vi "ControlArmInterface.vi"() -> ()   [LabVIEW 2024]
uses:
  <vilib>/Instr/_visa.llb/VISA Configure Serial Port (Instr).vi
panel:
  out "string":string
  in  "Power Button":bool
  in  "Position Maximum":bool
  in  "Position Minimum":bool
  in  "BackwardButton":bool
  in  "ForwardButton":bool
  in  "ScramButton":bool
  in  "SpeedSelectButton":bool
  in  "ElectormagnetButton":bool
  out "Analog In 4":u16(slide)=187 scale=0.0..1023.0
  out "Analog In 3":u16(slide)=187 scale=0.0..1023.0
  out "Analog In 2":u16(slide)=187 scale=0.0..1023.0
  out "Analog In 1":u16(knob)=187 scale=0.0..1023.0
  out "Digital Inputs 2":bool[](array[boolean])=[TRUE, TRUE, TRUE, TRUE, TRUE, TRUE, TRUE, TRUE]
  out "Digital Inputs":bool[](array[boolean])=[TRUE, TRUE, TRUE, TRUE, TRUE, TRUE, TRUE, TRUE]
  out "Hex data received":string
  in  "Send":bool
  in  "stop":bool
  in  "VISA resource name":refnum<visa-resource-name>
  # "Speed Select Bit"
  # "Scram Bit\nPower Bit\nMagnet Bit\nForward Bit\nBackward Bit\nMinimum Position \nMaximum Position\nMotor Active"
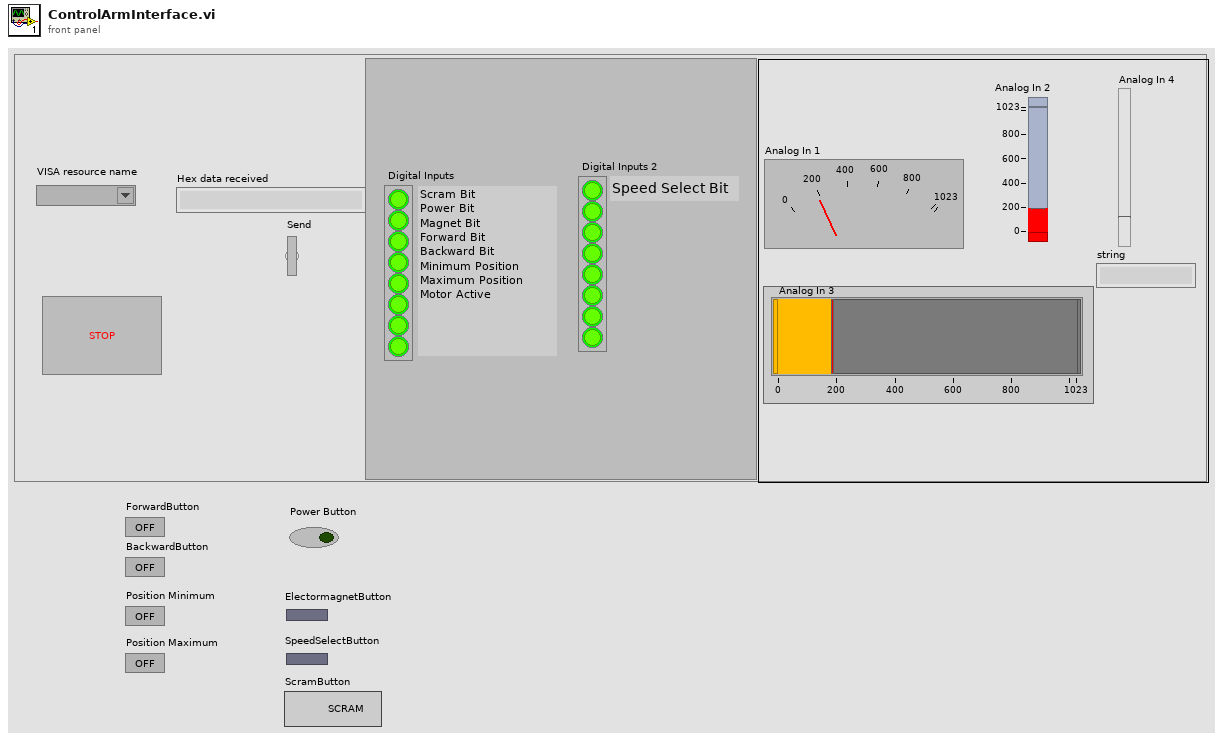
[diagram p1: front panel]
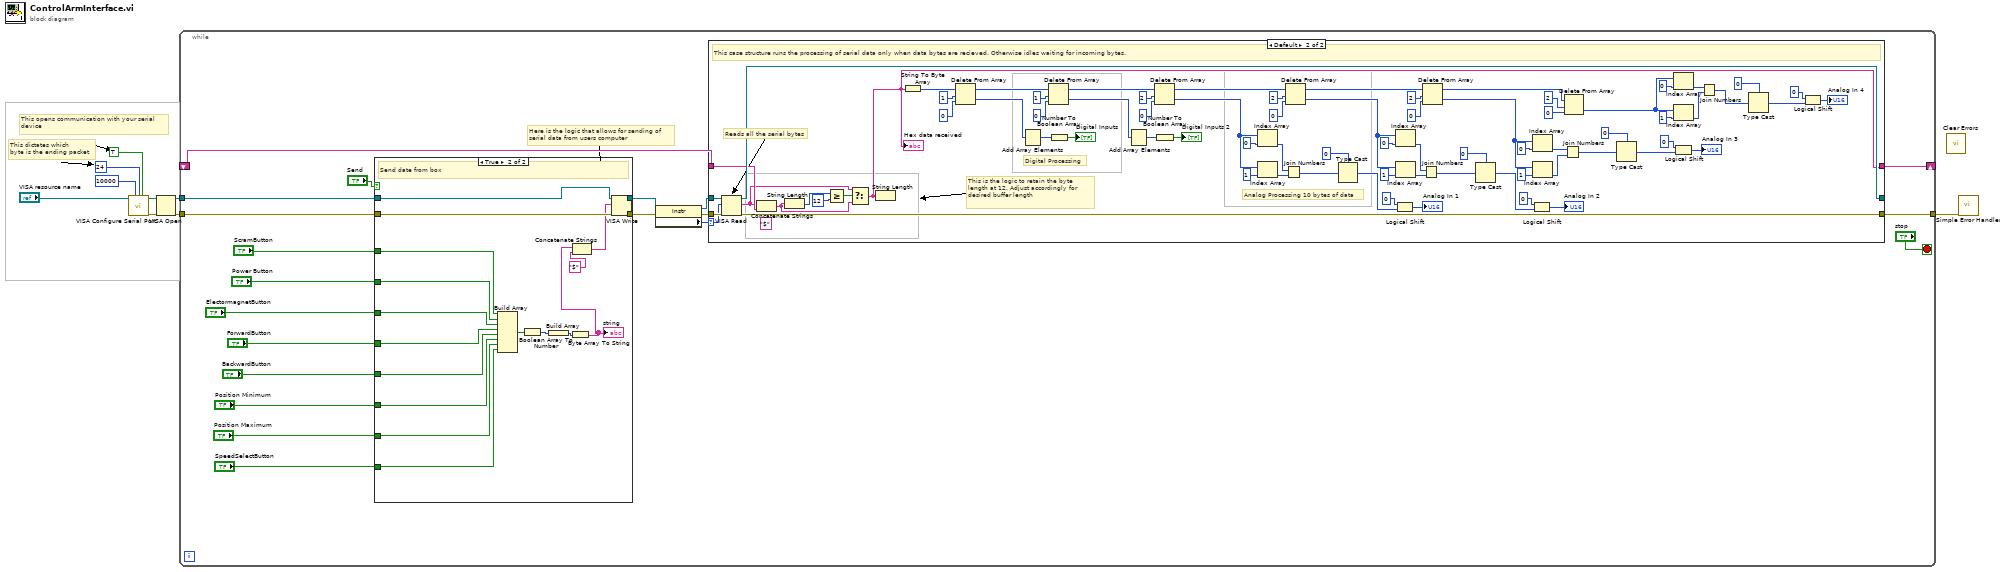
[diagram p0: block diagram]
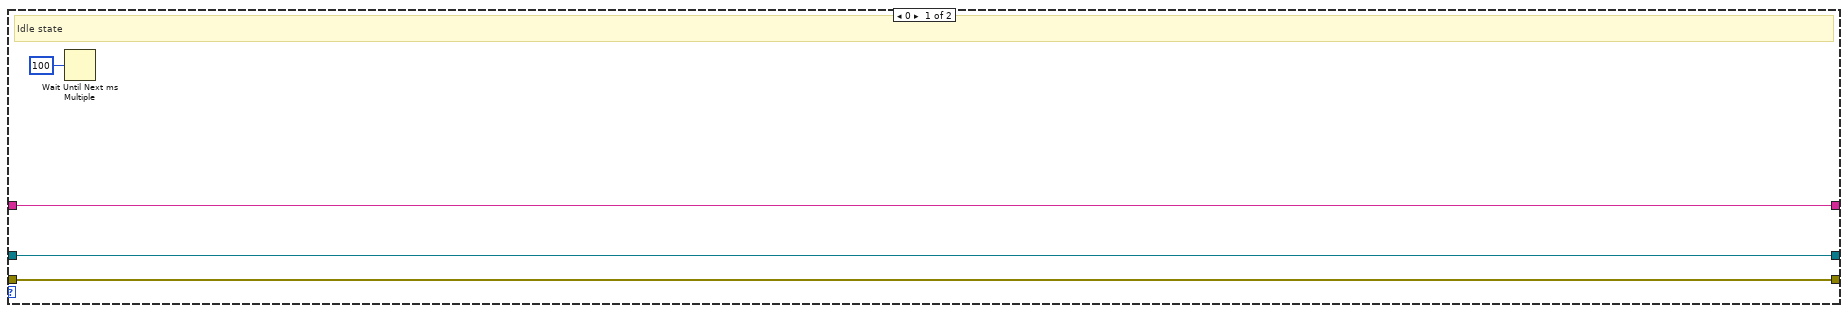
[diagram p2: hidden frame]
diagram:
  # "This dictates which\nbyte is the ending packet"
  # "This opens communication with your serial\ndevice"
  n1 = call-poly "VISA Configure Serial Port"("VISA resource name"="VISA resource name", "timeout (10sec)"=u32 10000, "termination char\n(0xA = '\\n' = LF)"=u8 24 ("termination char\n(0xA = '\\n' = LF)"), "Enable Termination\nChar (T)"=TRUE ("Enable Termination\nChar (T)")) -> ("VISA resource name out"=w5:refnum<visa-resource-name>, "error out"=w4:errorcluster)  [unwired: 10 in]
  n2 = VISA Open(error in (no error)=w4, VISA resource name=w5) -> (VISA resource name=w3:refnum<visa-resource-name>, error out=w2:errorcluster)  [unwired: 3 in]
  n3 = while {
    shift-right: [w22] -> _
    shift-left: _ -> [w21]
    tunnel: w3 -> [w20]
    tunnel: w2 -> [w19]
    tunnel: [w18] -> w1
    stop <- "stop" stop-if-true
    # "Here is the logic that allows for sending of \nserial data from users computer"
    n4 = case shown="True" "Send" {
      tunnel: [w111 w129] -> w27
      tunnel: w20 -> [w110 w128]
      tunnel: w19 -> [w111 w127]
      tunnel: [w110 w126] -> w28
      tunnel: "Power Button" -> [_ w122]
      tunnel: "Position Maximum" -> [_ w121]
      tunnel: "Position Minimum" -> [_ w120]
      tunnel: "BackwardButton" -> [_ w119]
      tunnel: "ForwardButton" -> [_ w118]
      tunnel: "ScramButton" -> [_ w117]
      tunnel: "SpeedSelectButton" -> [_ w116]
      tunnel: "ElectormagnetButton" -> [_ w115]
      frame False {
        # "Idle State"
      }
      frame True {
        # "Send date from box"
        n5 = Build Array(w117, w122, w115, w118, w119, w120, w121, w116) -> (w123:bool[])
        n6 = Boolean Array To Number(Boolean array=w123) -> (number=w124:u32)
        n7 = Build Array(w124) -> (w125:u32[])
        n8 = Byte Array To String(unsigned byte array=w125) -> (string=w114:string)
        "string" <- w114
        n9 = Concatenate Strings "Concatenate Strings"(w114, "$" ("element")) -> (w112:string)
        n10 = VISA Write(VISA resource name=w128, write buffer=w112, error in (no error)=w127) -> (VISA resource name out=w126:refnum<visa-resource-name>, error out=w129:errorcluster)  [unwired: 1 out]
      }
    }
    n11 = property class="Instr"(reference=w28, error in=w27) -> (reference out=w26:refnum<visa-resource-name>, error out=w25:errorcluster, "Serial Settings:Number of Bytes at Serial Port"=w23:u32)
    n12 = case shown="Default" w23 {
      selector: w23 -> [_ w105]
      tunnel: [w33 w109] -> _
      tunnel: [w32 w108] -> w18
      tunnel: w26 -> [w33 w107]
      tunnel: w25 -> [w32 w106]
      tunnel: w21 -> [w30 w104]
      tunnel: [w30 w92] -> w22
      frame 0 {
        # "Idle state"
        n13 = Wait Until Next ms Multiple(millisecond multiple=u32 100 ("millisecond timer value")) -> ()  [unwired: 1 out]
      }
      frame Default {
        (unwired) "$"
        # "Analog Processing 10 bytes of data"
        # "Digital Processing"
        # "This is the logic to retain the byte length at 12. Adjust accordingly for \ndesired buffer length"
        # "Reads all the serial bytes"
        # "This case structure runs the processing of serial data only when data bytes are recieved. Otherwise idles waiting for incoming bytes."
        n14 = VISA Read(VISA resource name=w107, byte count=w105, error in (no error)=w106) -> (VISA resource name out=w109:refnum<visa-resource-name>, read buffer=w100:string, error out=w108:errorcluster)  [unwired: 1 out]
        n15 = Concatenate Strings(w100, w104) -> (w99:string)
        n16 = String Length(string=w99) -> (length=w103:i32)
        n17 = Greater Or Equal?(x=w103, y=12) -> (x >= y?=w101:bool)
        n18 = Select(t=w100, s=w101, f=w99) -> (s? t:f=w92:string)
        "Hex data received" <- w92
        n19 = String Length(string=w92) -> ()  [unwired: 1 out]
        n20 = String To Byte Array(string=w92) -> (unsigned byte array=w97:u8[])
        n21 = Delete From Array "Delete From Array"(array=w97, length=1, index=0) -> (deleted portion=w98:u8[], array with subset deleted=w88:u8[])
        n22 = Add Array Elements(numeric array=w98) -> (sum=w96:u8)
        n23 = Delete From Array "Delete From Array"(array=w88, length=1, index=0) -> (deleted portion=w89:u8[], array with subset deleted=w38:u8[])
        n24 = Number To Boolean Array(number=w96) -> (Boolean array=→"Digital Inputs":bool[])
        n25 = Add Array Elements(numeric array=w89) -> (sum=w86:u8)
        n26 = Delete From Array "Delete From Array"(array=w38, length=2, index=0) -> (deleted portion=w79:u8[], array with subset deleted=w37:u8[])
        n27 = Number To Boolean Array(number=w86) -> (Boolean array=→"Digital Inputs 2":bool[])
        n28 = Index Array(array=w79, index=0) -> (element=w76:u8)
        n29 = Index Array(array=w79, index=1) -> (element=w75:u8)
        n30 = Join Numbers(hi=w76, lo=w75) -> ((hi.lo)=w74:u16)
        n31 = Delete From Array "Delete From Array"(array=w37, length=2, index=0) -> (deleted portion=w68:u8[], array with subset deleted=w36:u8[])
        n32 = Type Cast(type=u16 0 ("y"), x=w74) -> (*(type *) &x=w83:u16)
        n33 = Logical Shift(y=i16 0, x=w83) -> (x << y=→"Analog In 1":u16)
        n34 = Index Array(array=w68, index=0) -> (element=w71:u8)
        n35 = Index Array(array=w68, index=1) -> (element=w72:u8)
        n36 = Join Numbers(hi=w71, lo=w72) -> ((hi.lo)=w73:u16)
        n37 = Delete From Array "Delete From Array"(array=w36, length=2, index=0) -> (deleted portion=w55:u8[], array with subset deleted=w35:u8[])
        n38 = Type Cast(type=u16 0 ("y"), x=w73) -> (*(type *) &x=w64:u16)
        n39 = Logical Shift(y=i16 0, x=w64) -> (x << y=→"Analog In 2":u16)
        n40 = Index Array(array=w55, index=0) -> (element=w52:u8)
        n41 = Index Array(array=w55, index=1) -> (element=w51:u8)
        n42 = Join Numbers(hi=w52, lo=w51) -> ((hi.lo)=w50:u16)
        n43 = Delete From Array "Delete From Array"(array=w35, length=2, index=0) -> (deleted portion=w45:u8[])  [unwired: 1 out]
        n44 = Type Cast(type=u16 0 ("y"), x=w50) -> (*(type *) &x=w59:u16)
        n45 = Logical Shift(y=i16 0, x=w59) -> (x << y=→"Analog In 3":u16)
        n46 = Index Array(array=w45, index=0) -> (element=w47:u8)
        n47 = Index Array(array=w45, index=1) -> (element=w48:u8)
        n48 = Join Numbers(hi=w47, lo=w48) -> ((hi.lo)=w49:u16)
        n49 = Type Cast(type=u16 0 ("y"), x=w49) -> (*(type *) &x=w41:u16)
        n50 = Logical Shift(y=i16 0, x=w41) -> (x << y=→"Analog In 4":u16)
      }
    }
  }
  n51 = call <vilib>:"Clear Errors.vi"() -> ()  [unwired: 6 in, 2 out]
  n52 = call <vilib>:"Simple Error Handler.vi"("error in (no error)"=w1) -> ()  [unwired: 4 in, 5 out]
